vi "read help.vi"(8 "error in":errorcluster, 11 ".NET Refnum in":refnum<k24>) -> (0 "error out":errorcluster, 2 "Help":T1)   [LabVIEW 2015, in "Configuration Tool.lvlib"]
uses:
  Configuration Tool.lvlib
  XML Controls/help.ctl
  XML Controls/Path Cluster.ctl
  NationalInstruments.VeriStand.XMLReader
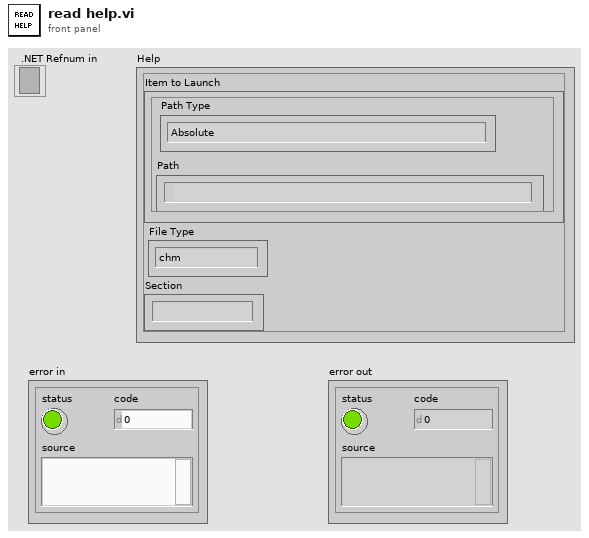
[diagram p1: front panel]
types:
  T1 = typedef "Configuration Tool.lvlib/help.ctl" = cluster{"Item to Launch":T2, "Section":string, "File Type":enum16{"chm", "other"}}
  T2 = typedef "Configuration Tool.lvlib/Path Cluster.ctl" = cluster{"Path":path, "Path Type":enum16{"Absolute", "To Base", "To Common Doc Dir", "To Application Data Dir"}}
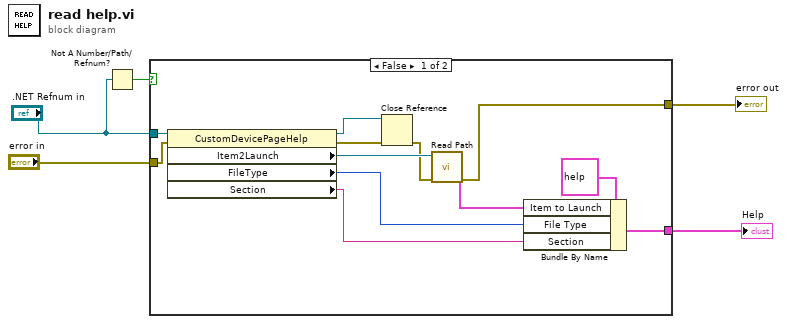
[diagram p0: block diagram]
diagram:
  n1 = Not A Number/Path/Refnum?(number/path/refnum=".NET Refnum in") -> (NaN/Path/Refnum?=w2:bool)
  n2 = case shown="False" w2 {
    tunnel: [w17 _] -> w5
    tunnel: ".NET Refnum in" -> [w15 _]
    tunnel: "error in" -> [w12 w18]
    tunnel: [w9 w18] -> w3
    frame False {
      n3 = property class="CustomDevicePageHelp"(reference=w15, error in=w12) -> (reference out=w14:refnum<k24>, error out=w13:errorcluster, "Item2Launch"=w11:refnum<k24>, "FileType"=w7:i32, "Section"=w6:string)
      n4 = Close Reference(reference=w14, error in (no error)=w13) -> (error out=w10:errorcluster)
      n5 = call "Read Path.vi"("error in (no error)"=w10, "Path Ref"=w11) -> ("error out"=w9:errorcluster, "Path"=w8:T2)  [unwired: 8 in]
      n6 = Bundle By Name(cluster=T1 {"Item to Launch"={"Path"=path "", "Path Type"=enum."Absolute"}, "Section"="", "File Type"=enum."chm"} ("Help"), "Item to Launch"=w8, "File Type"=w7, "Section"=w6) -> (w17:T1)
    }
    frame True {
    }
  }
  "Help" <- w5
  "error out" <- w3
